vi "Last1.vi"() -> ()   [LabVIEW 2020]
doc: "Use this template to build a producer/consumer design pattern. Use this template when you need to execute a process, such as data analysis, when a data source, such as a triggered acquisition, produces data at an uneven rate and you need to execute the process when the data becomes available."
uses:
  <vilib>/Utility/error.llb/DialogType.ctl
  <vilib>/DAQmx/read.llb/DAQmx Read (Analog Wfm 1Chan NSamp).vi
  <vilib>/DAQmx/create/channels.llb/DAQmx Create Channel (AI-Voltage-Basic).vi
  <vilib>/DAQmx/configure/timing.llb/DAQmx Timing (Sample Clock).vi
  <vilib>/Analysis/0measdsp.llb/Scaled Time Domain Window (DBL).vi
  <vilib>/DAQmx/miscellaneous.llb/DAQmx Fill In Error Info.vi
  <vilib>/Analysis/NI_AALPro.lvlib
panel:
  in  "Sample per Channel":dbl
  out "Frequency Peak":dbl format="%0.4f"
  in  "Filename":path=path "C:/Users/Hung/Desktop/TestSave.tdms"
  out "Record Signal":waveform(dbl)(graph)
  in  "Compare":dbl
  in  "Saving":bool
  out "RMS":dbl
  out "Numeric 2":i32
  out "Numeric":i32
  out "Waveform Graph":waveform(dbl)(graph)
  out "Data (Consumer Loop)":dbl[](array[numeric])
  in  "stop":bool
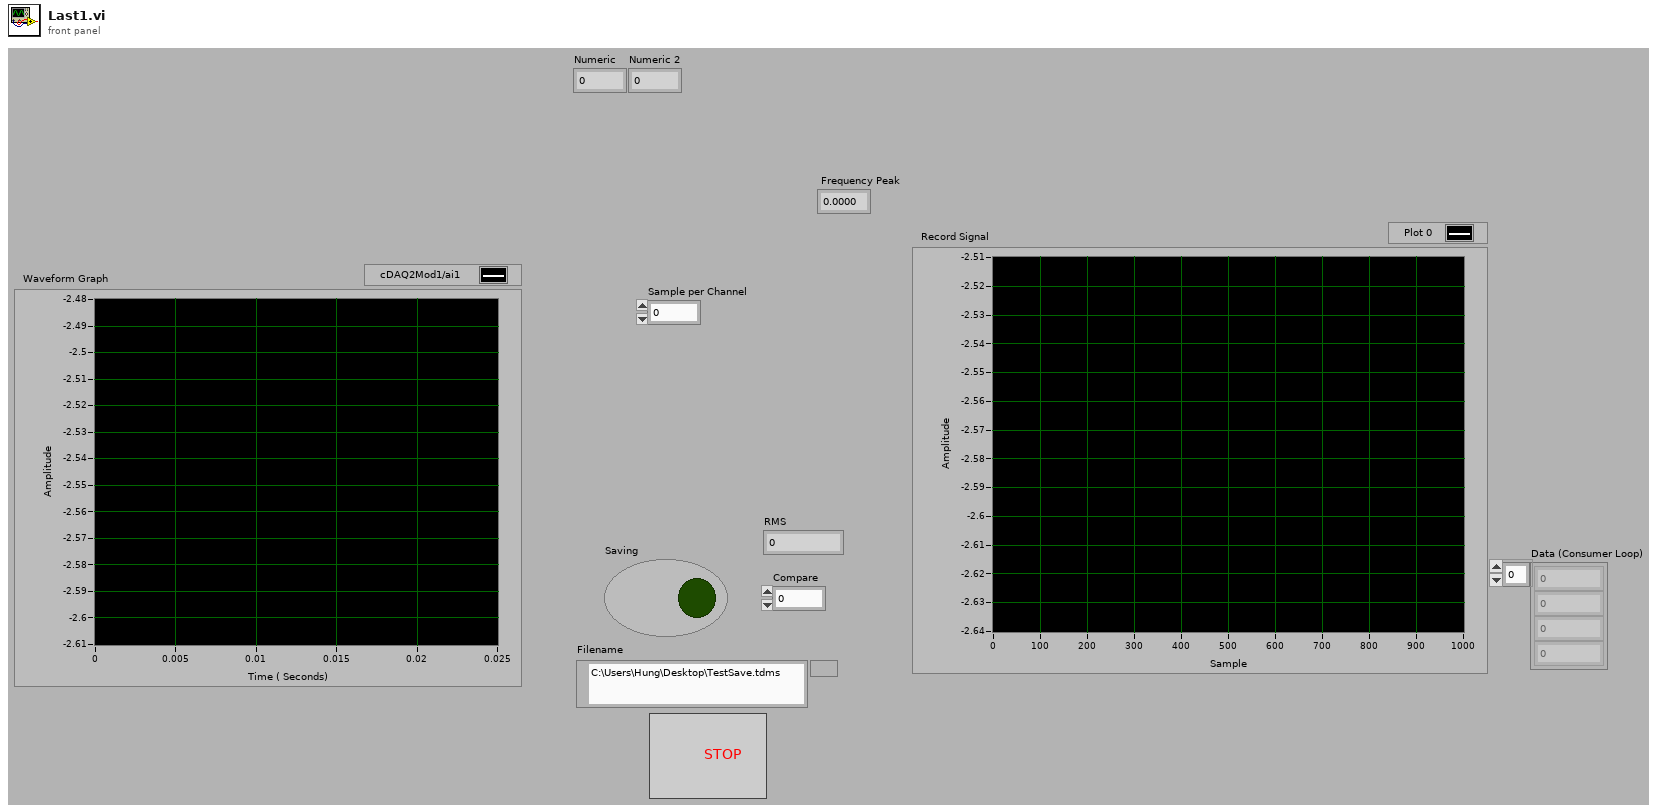
[diagram p1: front panel]
types:
  T1 = typedef "DialogType.ctl" = u16
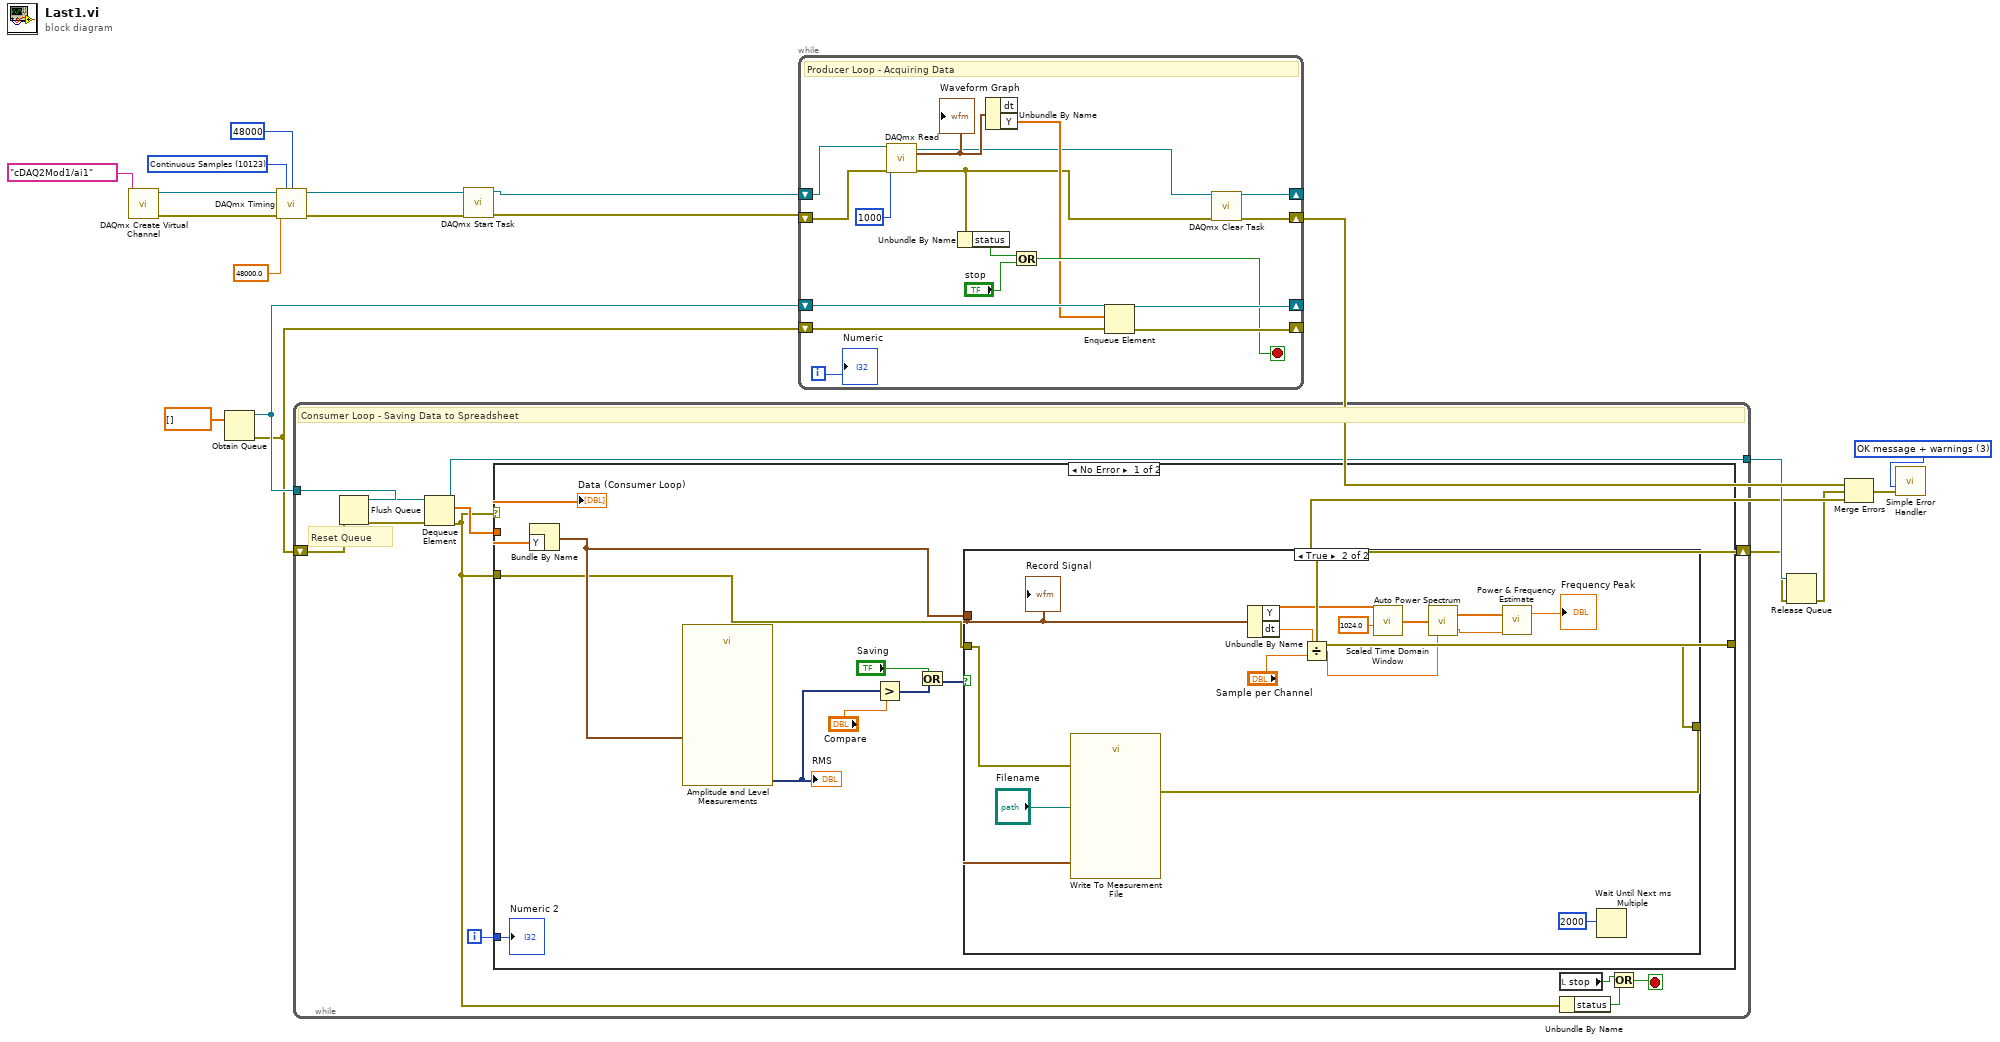
[diagram p0: block diagram]
diagram:
  w13 = 10123 items=["Finite Samples"=10178, "Continuous Samples"=10123, "Hardware Timed Single Point"=12522] ("sample mode")
  w20 = T1 3 items=["no dialog", "OK message", "continue or stop message", "OK message + warnings", "continue/stop + warnings"] ("type of dialog (OK msg:1)")
  n1 = call-poly <vilib>:"DAQmx Create Virtual Channel.vi"("physical channels"=tag "cDAQ2Mod1/ai1") -> ("task out"=w15:refnum<k21>, "error out"=w14:errorcluster)  [unwired: 13 in]
  n2 = Obtain Queue(element data type=dbl[] []) -> (queue out=w21:refnum<queue>, error out=w17:errorcluster)  [unwired: 3 in, 2 out]
  n3 = call-poly <vilib>:"DAQmx Timing.vi"("task/channels in"=w15, "sample mode"=w13, "samples per channel"=48000, "rate"=48000.0, "error in"=w14) -> ("task out"=w11:refnum<k21>, "error out"=w10:errorcluster)  [unwired: 9 in]
  n4 = while {
    tunnel: w21 -> [w25]
    shift-right: [w33] -> w2
    shift-left: w17 -> [w23]
    tunnel: [w26] -> w3
    i -> [w27]
    stop <- w29 stop-if-true
    # "Reset Queue"
    # "Consumer Loop - Saving Data to Spreadsheet"
    n5 = Flush Queue(queue=w25, error in (no error)=w23) -> (queue out=w24:refnum<queue>, error out=w22:errorcluster)  [unwired: 1 out]
    n6 = Dequeue Element(queue=w24, error in (no error)=w22) -> (queue out=w26:refnum<queue>, element=w32:dbl[], error out=w28:errorcluster)  [unwired: 2 out]
    n7 = case shown="No Error" w28 {
      tunnel: w32 -> [w36 _]
      tunnel: [w34 w59] -> w33
      tunnel: w28 -> [w35 w59]
      tunnel: w27 -> [w38 _]
      frame No Error {
        n8 = Bundle By Name("Y"=w36) -> (w37:waveform(dbl))  [unwired: 1 in]
        n9 = call "Amplitude and Level Measurements"("Signals"=w37) -> ("RMS"=w43:dynamicdata)  [unwired: 12 in, 2 out]
        "RMS" <- w43
        n10 = Greater?(x=w43, y="Compare") -> (0:w42:dynamicdata)
        n11 = Or(x="Saving", y=w42) -> (x .or. y?=w40:dynamicdata)
        n12 = case shown="True" w40 {
          tunnel: w37 -> [_ w57]
          tunnel: w35 -> [w44 w48]
          tunnel: [w44 w47] -> w34
          frame False {
          }
          frame True {
            n13 = call "Write To Measurement File"("Signals"=w57, "error in (no error)"=w48, "Filename"="Filename") -> ("error out"=w47:errorcluster)  [unwired: 14 in, 2 out]
            n14 = Unbundle By Name(w57) -> ("Y"=w56:dbl[], "dt"=w46:dbl)
            n15 = Divide(x=w46, y="Sample per Channel") -> (x/y=w49:dbl)
            n16 = call-poly <vilib>:"Scaled Time Domain Window.vi"("window parameter"=1024.0, "X"=w56) -> ("Windowed X"=w55:dbl[])  [unwired: 1 in, 8 out]
            n17 = call <vilib>:"Auto Power Spectrum.vi"("dt"=w49, "Signal (V)"=w55) -> ("df"=w54:dbl, "Power Spectrum (V^2 rms)"=w51:dbl[])
            n18 = call <vilib>:"Power & Frequency Estimate.vi"("df"=w54, "Power Spectrum (V^2 rms)"=w51) -> ("est frequency peak"=→"Frequency Peak":dbl)  [unwired: 3 in, 2 out]
            n19 = Wait Until Next ms Multiple(millisecond multiple=u32 2000 ("milliseconds to wait")) -> ()  [unwired: 1 out]
            "Record Signal" <- w57
          }
        }
        "Data (Consumer Loop)" <- w36
        "Numeric 2" <- w38
      }
      frame Error {
      }
    }
    n20 = local read "stop"() -> (w31:bool)
    n21 = Unbundle By Name(w28) -> ("status"=w30:bool)
    n22 = Or(x=w31, y=w30) -> (x .or. y?=w29:bool)
  }
  n23 = call <vilib>:"DAQmx Start Task.vi"("task/channels in"=w11, "error in"=w10) -> ("task out"=w8:refnum<k21>, "error out"=w7:errorcluster)  [unwired: 12 in]
  n24 = while {
    shift-right: [w71] -> _
    shift-left: w17 -> [w72]
    shift-right: [w73] -> _
    shift-left: w21 -> [w74]
    shift-right: [w63] -> w6
    shift-left: w8 -> [w67]
    shift-right: [w62] -> w5
    shift-left: w7 -> [w66]
    i -> [w61]
    stop <- w68 stop-if-true
    # "Producer Loop - Acquiring Data"
    n25 = call-poly <vilib>:"DAQmx Read.vi"("task/channels in"=w67, "number of samples per channel"=1000, "error in"=w66) -> ("task out"=w63:refnum<k21>, "data"=w64:waveform(dbl), "error out"=w62:errorcluster)  [unwired: 10 in]
    "Waveform Graph" <- w64
    n26 = Unbundle By Name(w62) -> ("status"=w70:bool)
    n27 = Unbundle By Name(w64) -> ("Y"=w65:dbl[])  [unwired: 1 out]
    n28 = Or(x=w70, y="stop") -> (x .or. y?=w68:bool)
    n29 = Enqueue Element(queue=w74, element=w65, error in (no error)=w72) -> (queue out=w73:refnum<queue>, error out=w71:errorcluster)  [unwired: 2 out]
    "Numeric" <- w61
  }
  n30 = call <vilib>:"DAQmx Clear Task.vi"("task in"=w6, "error in"=w5) -> ("error out"=w18:errorcluster)  [unwired: 13 out]
  n31 = Release Queue(queue=w3, error in (no error)=w2) -> (error out=w1:errorcluster)  [unwired: 1 in, 2 out]
  n32 = Merge Errors(w18, w1, w2) -> (w19:errorcluster)
  n33 = call <vilib>:"Simple Error Handler.vi"("type of dialog (OK msg:1)"=w20, "error in (no error)"=w19) -> ()  [unwired: 8 out]
